vi "Read from DAshboard.vi"() -> (3 "output cluster":T1)   [LabVIEW 2017]
uses:
  <vilib>/Rock Robotics/Network Tables/NT Read Number.vi
panel:
  out "Speed Rate":dbl
  out "Speed Deadband":dbl
  out "Turning Rate":dbl
  out "Turning Deadband":dbl
  out "Climb Time":dbl
  out "Climb Setpoint":dbl
  out "Button Lower Arm Time":dbl
  out "Button Lower Arm Setpoint":dbl
  out "Button Lift Arm Time":dbl
  out "Button Lift Arm Setpoint":dbl
  out "Release Time":dbl
  out "Release Setpoint":dbl
  out "Grab Time":dbl
  out "Grab Setpoint":dbl
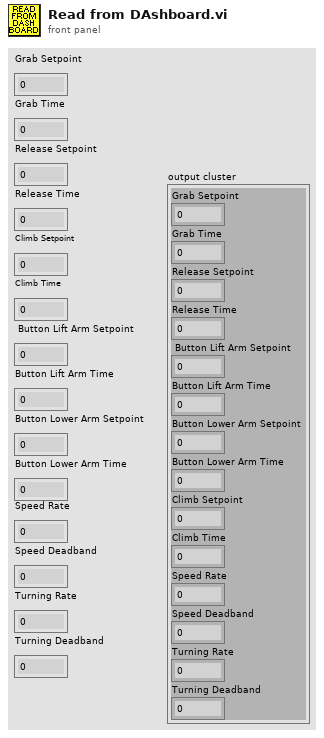
[diagram p1: front panel]
types:
  T1 = cluster{"Grab Setpoint ":dbl, "Grab Time ":dbl, "Release Setpoint ":dbl, "Release Time ":dbl, " Button Lift Arm Setpoint ":dbl, "Button Lift Arm Time ":dbl, "Button Lower Arm Setpoint ":dbl, "Button Lower Arm Time ":dbl, "Climb Setpoint ":dbl, "Climb Time ":dbl, "Speed Rate ":dbl, "Speed Deadband ":dbl, "Turning Rate ":dbl, "Turning Deadband ":dbl}
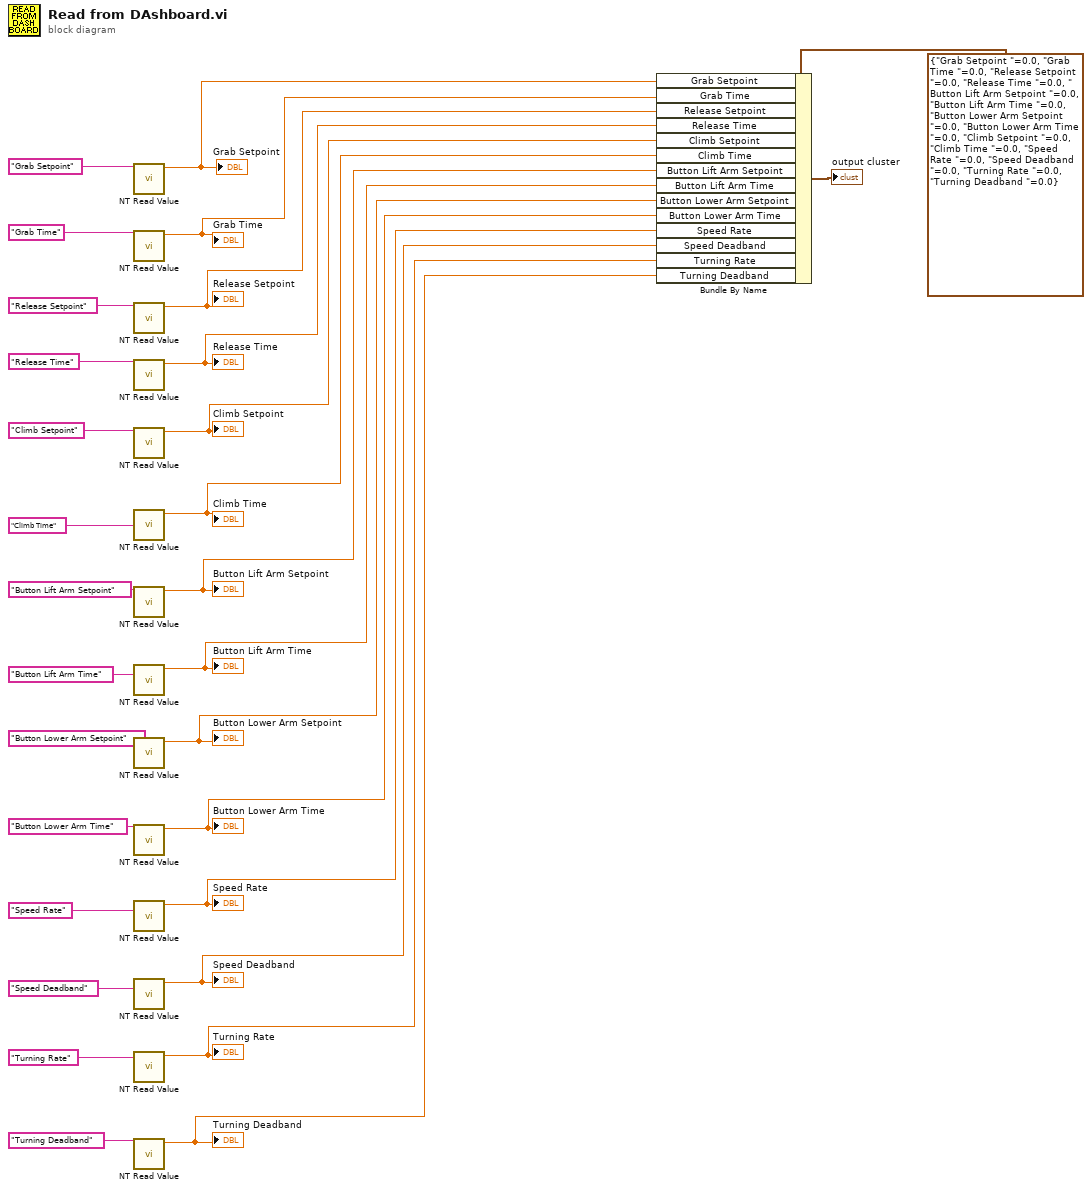
[diagram p0: block diagram]
diagram:
  n1 = call-poly <vilib>:"NT Read Value.vi"("Name"="Grab Setpoint") -> ("Numeric"=w3:dbl)  [unwired: 9 in, 1 out]
  "Grab Setpoint" <- w3
  n2 = call-poly <vilib>:"NT Read Value.vi"("Name"="Grab Time") -> ("Numeric"=w14:dbl)  [unwired: 9 in, 1 out]
  "Grab Time" <- w14
  n3 = call-poly <vilib>:"NT Read Value.vi"("Name"="Release Setpoint") -> ("Numeric"=w16:dbl)  [unwired: 9 in, 1 out]
  "Release Setpoint" <- w16
  n4 = call-poly <vilib>:"NT Read Value.vi"("Name"="Release Time") -> ("Numeric"=w15:dbl)  [unwired: 9 in, 1 out]
  "Release Time" <- w15
  n5 = call-poly <vilib>:"NT Read Value.vi"("Name"="Climb Setpoint") -> ("Numeric"=w13:dbl)  [unwired: 9 in, 1 out]
  "Climb Setpoint" <- w13
  n6 = call-poly <vilib>:"NT Read Value.vi"("Name"="Climb Time") -> ("Numeric"=w12:dbl)  [unwired: 9 in, 1 out]
  "Climb Time" <- w12
  n7 = call-poly <vilib>:"NT Read Value.vi"("Name"="Button Lift Arm Setpoint") -> ("Numeric"=w11:dbl)  [unwired: 9 in, 1 out]
  "Button Lift Arm Setpoint" <- w11
  n8 = call-poly <vilib>:"NT Read Value.vi"("Name"="Button Lift Arm Time") -> ("Numeric"=w10:dbl)  [unwired: 9 in, 1 out]
  "Button Lift Arm Time" <- w10
  n9 = call-poly <vilib>:"NT Read Value.vi"("Name"="Button Lower Arm Setpoint") -> ("Numeric"=w9:dbl)  [unwired: 9 in, 1 out]
  "Button Lower Arm Setpoint" <- w9
  n10 = call-poly <vilib>:"NT Read Value.vi"("Name"="Button Lower Arm Time") -> ("Numeric"=w8:dbl)  [unwired: 9 in, 1 out]
  "Button Lower Arm Time" <- w8
  n11 = call-poly <vilib>:"NT Read Value.vi"("Name"="Speed Rate") -> ("Numeric"=w7:dbl)  [unwired: 9 in, 1 out]
  "Speed Rate" <- w7
  n12 = call-poly <vilib>:"NT Read Value.vi"("Name"="Speed Deadband") -> ("Numeric"=w6:dbl)  [unwired: 9 in, 1 out]
  "Speed Deadband" <- w6
  n13 = call-poly <vilib>:"NT Read Value.vi"("Name"="Turning Rate") -> ("Numeric"=w5:dbl)  [unwired: 9 in, 1 out]
  "Turning Rate" <- w5
  n14 = call-poly <vilib>:"NT Read Value.vi"("Name"="Turning Deadband") -> ("Numeric"=w4:dbl)  [unwired: 9 in, 1 out]
  "Turning Deadband" <- w4
  n15 = Bundle By Name(cluster=T1 {"Grab Setpoint "=0.0, "Grab Time "=0.0, "Release Setpoint "=0.0, "Release Time "=0.0, " Button Lift Arm Setpoint "=0.0, "Button Lift Arm Time "=0.0, "Button Lower Arm Setpoint "=0.0, "Button Lower Arm Time "=0.0, "Climb Setpoint "=0.0, "Climb Time "=0.0, "Speed Rate "=0.0, "Speed Deadband "=0.0, "Turning Rate "=0.0, "Turning Deadband "=0.0}, "Grab Setpoint"=w3, "Grab Time"=w14, "Release Setpoint"=w16, "Release Time"=w15, "Climb Setpoint"=w13, "Climb Time"=w12, "Button Lift Arm Setpoint"=w11, "Button Lift Arm Time"=w10, "Button Lower Arm Setpoint"=w9, "Button Lower Arm Time"=w8, "Speed Rate"=w7, "Speed Deadband"=w6, "Turning Rate"=w5, "Turning Deadband"=w4) -> (→"output cluster":T1)
